vi "Calibrate xtal.vi"(5 "External Attenuation, dB":T8 format="%.2f", 7 "CART TCP Connection In":refnum<k5>, 8 "Error In":errorcluster, 9 "Max Input Power, dBm":T7 format="%.1f", 11 "RFSA Device":T16="RFSA") -> (0 "error out":errorcluster)   [LabVIEW 2012]
doc: "(c) Copyright 2006, National Instruments, Inc. This VI may not be duplicated, sold, or distributed without written consent from National Instruments."
uses:
  <userlib>/niRF/niSystem/SA/Includes/niSYS - RFSA - INC - STYP - Handle.ctl
  <userlib>/niRF/niSystem/SA/Includes/niSYS - SA - INC - STYP - Trigger.ctl
  <userlib>/niRF/niSystem/SA/Includes/niSYS - SA - INC - STYP - Trigger Delay.ctl
  <userlib>/niRF/niSystem/SA/Includes/niSYS - SA - INC - STYP - Timeout.ctl
  <userlib>/niRF/niBasic/SA/Spectrum/Includes/niBASIC - SA - Spectrum - INC - STYP - Averaging.ctl
  <userlib>/niRF/niBasic/SA/Spectrum/Includes/niBASIC - SA - Spectrum - INC - STYP - Measurement.ctl
  <userlib>/niRF/niSystem/SA/Includes/niSYS - SA - INC - STYP - Frequency Reference.ctl
  <userlib>/niRF/niSystem/SA/Includes/niSYS - SA - INC - STYP - External Attenuation.ctl
  <userlib>/niRF/niSystem/SA/Includes/niSYS - SA - INC - STYP - Max Input Power.ctl
  <userlib>/niRF/niSystem/SA/Includes/niSYS - SA - INC - STYP - Center Frequency.ctl
  <userlib>/niRF/niBasic/SA/Spectrum/Includes/niBASIC - SA - Spectrum - INC - STYP - FFT Window.ctl
  <userlib>/niRF/niBasic/SA/Spectrum/Includes/niBASIC - SA - Spectrum - INC - STYP - Measurement RBW.ctl
  <userlib>/niRF/niSystem/SA/Includes/niSYS - SA - INC - STYP - Span.ctl
  <userlib>/niRF/niBasic/SA/Spectrum/Includes/niBASIC - SA - Spectrum - INC - STYP - FFT Size.ctl
  <userlib>/niRF/niBasic/SA/Spectrum/Includes/niBASIC - SA - Spectrum - INC - STYP - Filter Type.ctl
  <userlib>/niRF/niSystem/SA/Includes/niSYS - SA - INC - STYP - Measurement Request.ctl
  <userlib>/niRF/niBasic/SA/Spectrum/Includes/niBASIC - SA - Spectrum - INC - STYP - Measurement Trace Type.ctl
panel:
  out "Array":string[](array[string])
  in  "Filter Type":T1
  in  "FFT Size":T2={"Auto"=enum."On", "Min Pnts/RBW"=3.1, "Window Length"=706, "FFT Length"=1024} {"Min Pnts/RBW" format="%.1f"}
  in  "Span, Hz":T3=1000000.0 format="%^.3e"
  in  "Measurement RBW, Hz":T4={"Auto"=enum."On", "RBW, Hz"=1000000.0} {"RBW, Hz" format="%^.3e"}
  in  "FFT Window":T5
  in  "RFSA Center Frequency, Hz":T6=5500000000.0 format="%^.6e"
  out "Spectrum Graph":T9(graph)={999501953.125, "Time Domain Interval, sec"=4882.8125, "Waveform Measurement Trace"=[-94.58885960127041, -96.86839023376476, -99.44994709212702, -95.73980201325817, -94.85468685558206, -93.89939819937095, -92.96907780368053, -94.62427677362473, -96.00114334271848, -95.0773520951145, -94.62079733063136, -95.66039665905808, -97.26831199401815, -94.4245843897965, -94.11636842862069, -93.58322383773326, -96.15404542236388, -96.24945397470107, -95.50507217914763, -96.54108841377801, -96.20009898290628, -94.5853296471187, -92.45746866418841, -91.28538347271048, -91.87185526400654, -94.56638317616594, -96.80701098668649, -98.3947929158942, -98.51183674015738, -97.19248581591714, -96.81596744977271, -95.42900485531823, -95.06526491233971, -94.58696887517611, -95.97070348701587, -96.12508871585825, -96.44070407370447, -95.79000716907146, -97.40271981045801, -96.56026806674593, -96.63105214105727, -95.37951512730523, -95.0709837906345, -97.57170348129546, -98.65428166191879, -92.85960027957853, -90.69744081914348, -91.78092902523147, -93.01528314210488, -94.00436029202501, -93.35100459361215, -93.65439480062977, -94.03853395069989, -94.46526514886557, -94.89042305851434, -94.67424970039717, -93.63794705250254, -92.45925730447641, -92.65908155014344, -93.60044471338867, -94.45278046002886, -94.14161306416081, -95.1968357622903, -94.78018101642988, -94.3521734655379, -93.66111421566106, -94.84863517357037, -94.5954023919716, -96.31573035476218, -96.10673186698642, -95.71535800929679, -94.23828099215436, -93.52563000159624, -95.57033866863337, -95.53015116793134, -93.56809331780974, -92.7606452725199, -93.57072573308072, -95.32780281550693, -92.86665354898099, -93.1370950166728, -94.12900193004297, -94.87833817452723, -94.72912032302605, -94.17479444496155, -94.72686892886344, -93.6596877329905, -92.66964149507194, -93.08938347771124, -94.20661112927449, -97.92818192608922, -94.73725815144995, -93.72795972831032, -95.83148845299667, -93.96304770180853, -93.50544784378508, -92.44166060977277, -93.27927003206689, -87.23502888503836, -72.11564523212036, -65.2815070033974, -63.751961771120435, -63.76202638288482, -64.94683436227825, -71.0137879230945, -85.10120059441533, -91.83446895184292, -90.61921828145796, -90.72235231920887, -91.03886336724534, -91.42747554368565, -91.50468859500515, -90.91036635524621, -91.23961076459484, -93.16256151029376, -95.66587614800164, -96.70895620214242, -94.44704301225457, -93.34996435212136, -92.18571998503167, -92.8876926563818, -93.5060742547249, -94.69941271506612, -97.92708620913864, -95.25428896670476, -92.62306680566677, -91.3874988202419, -91.85885903026352, -93.43215873965788, -94.90985702146794, -94.99607107512729, -94.53014477422813, -94.84999122998677, -95.93647533060847, -95.05672593509198, -97.64855424631322, -95.46215659926096, -94.67802340702697, -94.36305677166051, -95.093191185747, -95.15591730271399, -94.6393427453004, -95.01042716486224, -93.48932052409448, -93.1088259750116, -95.79379158863588, -94.27401403528606, -94.39185567902642, -95.78566610842289, -96.2278510846579, -97.35096719200405, -94.09028417116734, -93.67455962770373, -92.52661334344788, -92.28656403084389, -93.48717465263262, -95.87262940934153, -96.55075020577934, -96.23995801594376, -95.62432812173306, -95.53325913753295, -95.37316281463609, -96.84726282341614, -96.18759453809396, -92.65258606681302, -91.1549944641086, -91.18877556936353, -91.65922730189286, -92.7088197008887, -93.55252845804509, -93.23891521766758, -93.50579589024103, -93.22879114454076, -93.62878875149401, -94.89920966153908, -94.49841305989179, -94.31891446472981, -93.3315995436115, -92.9576487551588, -94.98762611566268, -97.76488288036198, -96.68686917193047, -95.69013350308543, -95.23811265655995, -95.43343805014592, -96.1176286234256, -98.40428345012647, -97.1939542411557, -93.8709557440311, -92.5732899687502, -93.19402090455232, -93.4806645014271, -92.62376136260087, -93.4169081651324, -95.1135305356191, -95.44327303741449, -95.97664612099189, -95.20918978347628, -93.30477056749844, -92.75514488033883, -92.92596032798458, -94.3147334729053, -95.75765916034278, -97.49920812243585, -93.12822887068018]}
  in  "Frequency Reference":T10={" Reference Source"=enum."On Board Clock", "Frequency, Hz"=10000000.0, "Backplane Source"=enum."None"} {"Frequency, Hz" format="%^.6e"}
  out "Spectrum Measurement":T11={"Peak Amplitude, dBm"=-63.751961771120435, "Peak Frequency, Hz"=999995117.1875, "Number of Points"=256, "Start Frequency, Hz"=999501953.125, "Space Frequency, Hz"=4882.8125} {"Space Frequency, Hz" format="%^.6e"; "Start Frequency, Hz" format="%^.6e"; "Peak Frequency, Hz" format="%^.6e"; "Peak Amplitude, dBm" format="%.2f"}
  in  "Spectrum Averaging":T12={"Averages"=10, "Average State"=enum."On", "Average Mode"=enum."Repeat", "Average Type"=enum."Log"}
  in  "Timeout, sec":T13=10.0 format="%.3f"
  in  "Trigger":T14={"Source"=enum."Immediate", "Edge"=enum."Rising", "Delay, sec"=0.0, "Level, dBm"=-20.0, "Min Quiet Time, sec"=0.0} {"Min Quiet Time, sec" format="%^.2e"; "Level, dBm" format="%.1f"; "Delay, sec" format="%^.2e"}
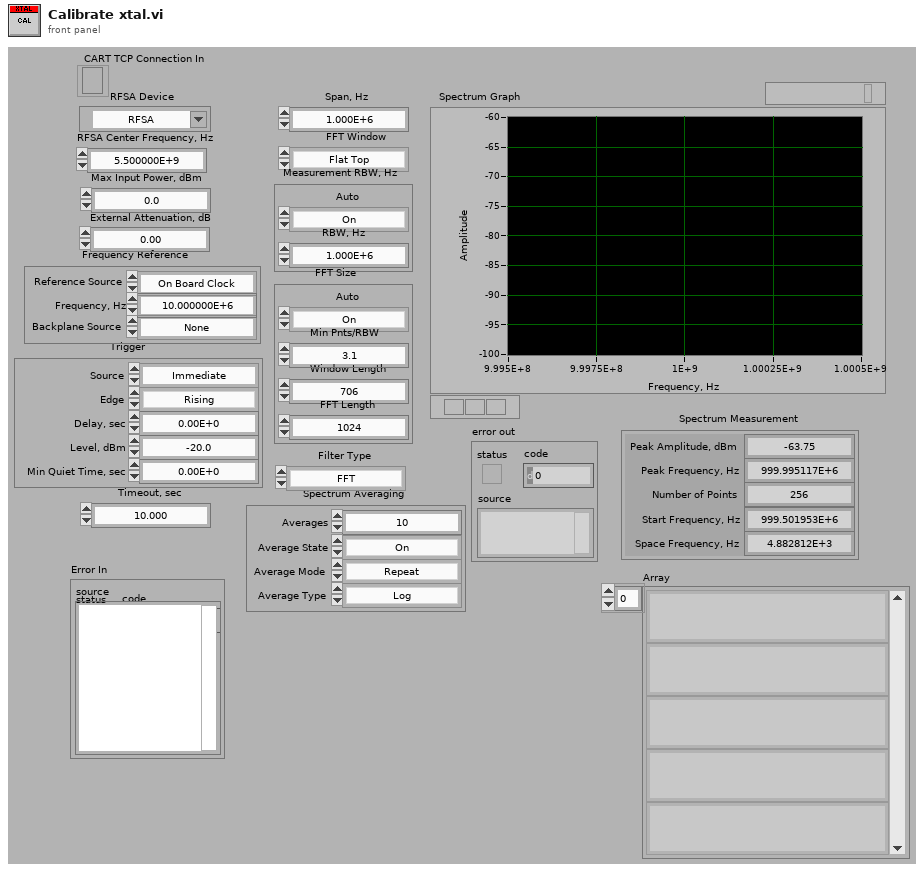
[diagram p1: front panel]
types:
  T1 = typedef "niBASIC - SA - Spectrum - INC - STYP - Filter Type.ctl" = enum16{"FFT", "5-Pole", "Gaussian"}
  T2 = typedef "niBASIC - SA - Spectrum - INC - STYP - FFT Size.ctl" = cluster{"Auto":enum16{"Off", "On"}, "Min Pnts/RBW":dbl, "Window Length":i32, "FFT Length":i32}
  T3 = typedef "niSYS - SA - INC - STYP - Span.ctl" = dbl
  T4 = typedef "niBASIC - SA - Spectrum - INC - STYP - Measurement RBW.ctl" = cluster{"Auto":enum16{"Off", "On"}, "RBW, Hz":dbl}
  T5 = typedef "niBASIC - SA - Spectrum - INC - STYP - FFT Window.ctl" = enum16{"Flat Top", "Uniform", "Hanning", "Hamming", "Gaussian", "Blackman", "Blackman-Harris", "Kaiser-Bessel 70 dB", "Kaiser-Bessel 90 dB", "Kaiser-Bessel 110 dB"}
  T6 = typedef "niSYS - SA - INC - STYP - Center Frequency.ctl" = dbl
  T7 = typedef "niSYS - SA - INC - STYP - Max Input Power.ctl" = dbl
  T8 = typedef "niSYS - SA - INC - STYP - External Attenuation.ctl" = dbl
  T9 = cluster{dbl, "Time Domain Interval, sec":dbl, "Waveform Measurement Trace":dbl[]}
  T10 = typedef "niSYS - SA - INC - STYP - Frequency Reference.ctl" = cluster{" Reference Source":enum16{"On Board Clock", "Ref In", "PXI Clock 10"}, "Frequency, Hz":dbl, "Backplane Source":enum16{"None", "Ref In", "On Board Clock"}}
  T11 = typedef "niBASIC - SA - Spectrum - INC - STYP - Measurement.ctl" = cluster{"Peak Amplitude, dBm":dbl, "Peak Frequency, Hz":dbl, "Number of Points":i32, "Start Frequency, Hz":dbl, "Space Frequency, Hz":dbl}
  T12 = typedef "niBASIC - SA - Spectrum - INC - STYP - Averaging.ctl" = cluster{"Averages":i32, "Average State":enum16{"Off", "On"}, "Average Mode":enum16{"Exponential", "Repeat"}, "Average Type":enum16{"RMS", "Log", "Scalar", "Max", "Min"}}
  T13 = typedef "niSYS - SA - INC - STYP - Timeout.ctl" = dbl
  T14 = typedef "niSYS - SA - INC - STYP - Trigger.ctl" = cluster{"Source":enum16{"Immediate", "External", "Software", "RTSI 0", "RTSI 1", "RTSI 2", "RTSI 3", "RTSI 4", "RTSI 5", "RTSI 6", "RTSI 7", "PFI 0", "PFI 1", "PFI 2", "PXI Star", "Power"}, "Edge":enum16{"Rising", "Falling"}, "Delay, sec":T15, "Level, dBm":dbl, "Min Quiet Time, sec":dbl}
  T15 = typedef "niSYS - SA - INC - STYP - Trigger Delay.ctl" = dbl
  T16 = typedef "niSYS - RFSA - INC - STYP - Handle.ctl" = refnum<k15>
  T17 = typedef "niBASIC - SA - Spectrum - INC - STYP - Measurement Handle.ctl" = refnum<notifier>
  T18 = typedef "niBASIC - SA - Spectrum - INC - STYP - Measurement Trace Type.ctl" = enum16{"Unprocessed I/Q", "Measurements", "Average Spectrum"}
  T19 = typedef "niSYS - SA - INC - STYP - Measurement Request.ctl" = enum16{"Measure", "Fetch", "Initiate"}
  T20 = typedef "niSYS - SA - INC - STYP - Measurement Trace.ctl" = dbl[]
  T21 = typedef "niSYS - SA - INC - STYP - Real Waveform.ctl" = cluster{"x0":dbl, "dx":dbl, "y":dbl[]}
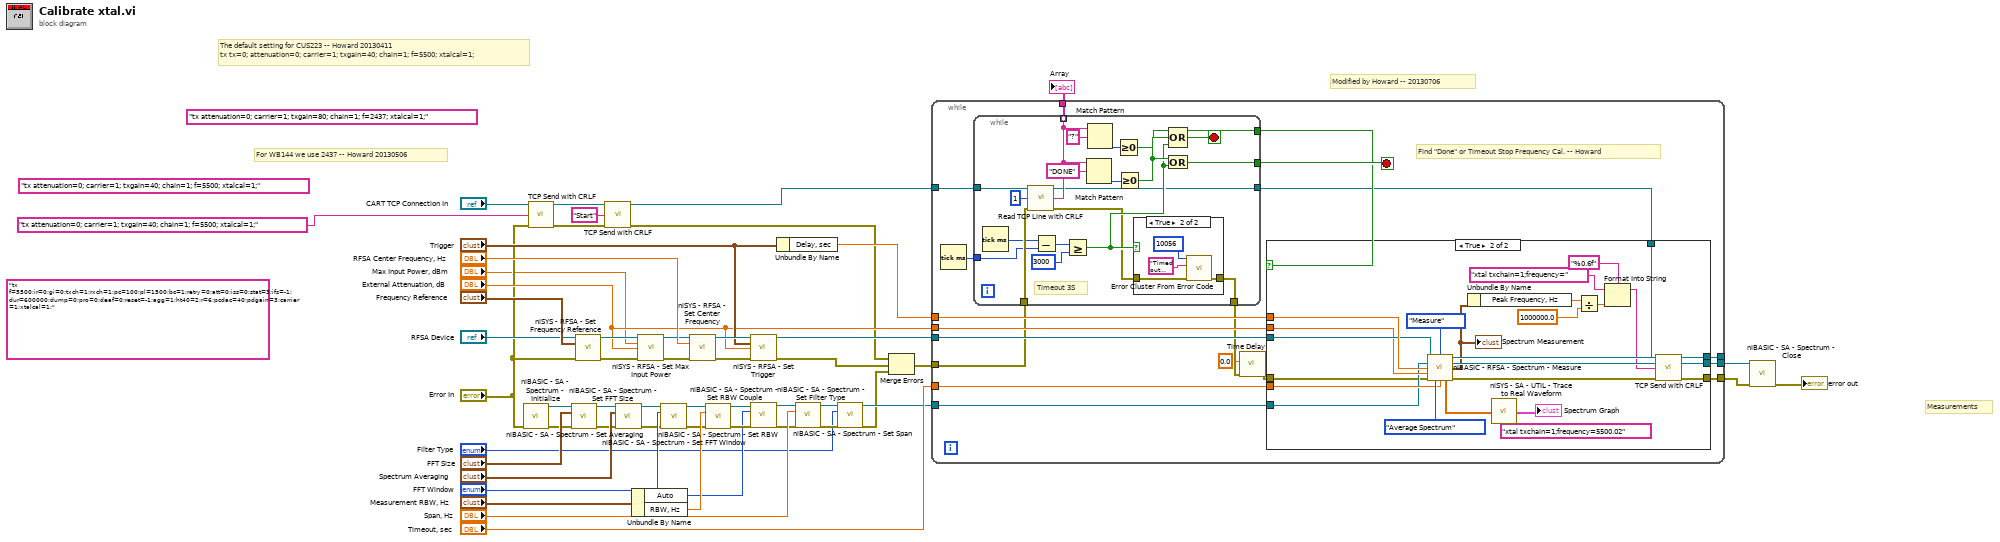
[diagram p0: block diagram]
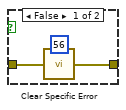
[diagram p2: hidden frame]
diagram:
  (unwired) "tx f=5500;ir=0;gi=0;txch=1;rxch=1;pc=100;pl=1500;bc=1;retry=0;att=0;iss=0;stat=3;ifs=-1;dur=600000;dump=0;pro=0;deaf=0;reset=-1;agg=1;ht40=2;r=6;pcdac=40;pdgain=3;carrier=1;xtalcal=1;"
  (unwired) "tx attenuation=0; carrier=1; txgain=40; chain=1; f=5500; xtalcal=1;" ("data in")
  (unwired) "tx attenuation=0; carrier=1; txgain=80; chain=1; f=2437; xtalcal=1;" ("data in")
  # "Modified by Howard -- 20130706"
  # "For WB144 we use 2437 -- Howard 20130506"
  # "The default setting for CUS223 -- Howard 20130411\ntx tx=0; attenuation=0; carrier=1; txgain=40; chain=1; f=5500; xtalcal=1;"
  # "Measurements"
  n1 = call <userlib>:"niBASIC - SA - Spectrum - Initialize.vi"("error in (no error)"="Error In") -> ("Measurement Handle Out"=w29:T17, "error out"=w30:errorcluster)  [unwired: 1 in, 12 out]
  n2 = call "TCP Send with CRLF.vi"("CART TCP Connection"="CART TCP Connection In", "data in"="tx attenuation=0; carrier=1; txgain=40; chain=1; f=5500; xtalcal=1;", "error IO"="Error In") -> ("CART TCP Connection Out"=w11:refnum<k5>, "error out"=w12:errorcluster)  [unwired: 11 in]
  n3 = call <userlib>:"niBASIC - SA - Spectrum - Set FFT Size.vi"("Measurement Handle In"=w29, "FFT Size"="FFT Size", "error in (no error)"=w30) -> ("Measurement Handle Out"=w43:T17, "error out"=w44:errorcluster)  [unwired: 11 out]
  n4 = call <userlib>:"niSYS - RFSA - Set Frequency Reference.vi"("RFSA Handle In"="RFSA Device", "Frequency Reference"="Frequency Reference", "error in (no error)"="Error In") -> ("RFSA Handle Out"=w32:T16, "error out"=w31:errorcluster)  [unwired: 1 in, 10 out]
  n5 = call "TCP Send with CRLF.vi"("CART TCP Connection"=w11, "data in"="Start", "error IO"=w12) -> ("CART TCP Connection Out"=w9:refnum<k5>, "error out"=w8:errorcluster)  [unwired: 11 in]
  n6 = call <userlib>:"niBASIC - SA - Spectrum - Set Averaging.vi"("Measurement Handle In"=w43, "Averaging"="Spectrum Averaging", "error in (no error)"=w44) -> ("Measurement Handle Out"=w41:T17, "error out"=w42:errorcluster)  [unwired: 11 out]
  n7 = Unbundle By Name("Measurement RBW, Hz") -> ("Auto"=w33:enum16{"Off", "On"}, "RBW, Hz"=w40:dbl)
  n8 = call <userlib>:"niSYS - RFSA - Set Max Input Power.vi"("RFSA Handle In"=w32, "Max Input Power, dBm"="Max Input Power, dBm", "External Attenuation, dB"="External Attenuation, dB", "error in (no error)"=w31) -> ("RFSA Handle Out"=w45:T16, "error out"=w46:errorcluster)  [unwired: 10 out]
  n9 = call <userlib>:"niBASIC - SA - Spectrum - Set FFT Window.vi"("Measurement Handle In"=w41, "FFT Window"="FFT Window", "error in (no error)"=w42) -> ("Measurement Handle Out"=w38:T17, "error out"=w39:errorcluster)  [unwired: 11 out]
  n10 = call <userlib>:"niSYS - RFSA - Set Center Frequency.vi"("RFSA Handle In"=w45, "RFSA Center Frequency, Hz"="RFSA Center Frequency, Hz", "error in (no error)"=w46) -> ("RFSA Handle Out"=w27:T16, "error out"=w28:errorcluster)  [unwired: 11 out]
  n11 = call <userlib>:"niBASIC - SA - Spectrum - Set RBW.vi"("Measurement Handle In"=w38, "RBW, Hz"=w40, "error in (no error)"=w39) -> ("Measurement Handle Out"=w35:T17, "error out"=w37:errorcluster)  [unwired: 11 out]
  n12 = call <userlib>:"niSYS - RFSA - Set Trigger.vi"("RFSA Handle In"=w27, "Trigger"="Trigger", "External Attenuation, dB"="External Attenuation, dB", "error in (no error)"=w28) -> ("RFSA Handle Out"=w24:T16, "error out"=w19:errorcluster)  [unwired: 10 out]
  n13 = call <userlib>:"niBASIC - SA - Spectrum - Set RBW Couple.vi"("Measurement Handle In"=w35, "Auto"=w33, "error in (no error)"=w37) -> ("Measurement Handle Out"=w34:T17, "error out"=w36:errorcluster)  [unwired: 11 out]
  n14 = Unbundle By Name("Trigger") -> ("Delay, sec"=w25:T15)
  n15 = call <userlib>:"niBASIC - SA - Spectrum - Set Span.vi"("Measurement Handle In"=w34, "Span, Hz"="Span, Hz", "error in (no error)"=w36) -> ("Measurement Handle Out"=w18:T17, "error out"=w16:errorcluster)  [unwired: 11 out]
  n16 = call <userlib>:"niBASIC - SA - Spectrum - Set Filter Type.vi"("Measurement Handle In"=w18, "Filter Type"="Filter Type", "error in (no error)"=w16) -> ("Measurement Handle Out"=w17:T17, "error out"=w15:errorcluster)  [unwired: 10 in, 1 out]
  n17 = Merge Errors(w8, w19, w15) -> (w7:errorcluster)
  n18 = while {
    tunnel: w25 -> [w71]
    tunnel: w24 -> [w70]
    tunnel: "External Attenuation, dB" -> [w69]
    tunnel: "Timeout, sec" -> [w68]
    tunnel: [w67] -> _
    tunnel: [w64] -> w4
    tunnel: [w66] -> w21
    tunnel: w17 -> [w65]
    tunnel: w9 -> [w63]
    tunnel: w7 -> [w62]
    tunnel: [w57] -> w3
    stop <- w61 stop-if-true
    # "Find \"Done\" or Timeout Stop Frequency Cal. -- Howard"
    n19 = Tick Count (ms)() -> (millisecond timer value=w58:u32)
    n20 = while {
      tunnel: w63 -> [w86]
      tunnel: w62 -> [w85]
      tunnel: [w79] -> w61
      tunnel: [w76] -> w60
      tunnel: [w75] -> w59
      tunnel: w58 -> [w74]
      tunnel: [w73] -> w57 mode=indexing
      tunnel: [w72] -> w56
      stop <- w81 stop-if-true
      # "Timeout 3S"
      n21 = Tick Count (ms)() -> (millisecond timer value=w84:u32)
      n22 = call "Read TCP Line with CRLF.vi"("TCP Connection In"=w86, "timeout ms (100)"=1, "error in"=w85) -> ("TCP Connection Out"=w72:refnum<k5>, "TCP Line"=w73:string, "error out"=w77:errorcluster)  [unwired: 10 in]
      n23 = Subtract(x=w84, y=w74) -> (x-y=w83:u32)
      n24 = Greater Or Equal?(x=w83, y=u32 3000) -> (x >= y?=w78:bool)
      n25 = Match Pattern(string=w73, regular expression="DONE") -> (offset past match=w91:i32)  [unwired: 1 in, 3 out]
      n26 = Match Pattern(string=w73, regular expression="?") -> (offset past match=w90:i32)  [unwired: 1 in, 3 out]
      n27 = Greater Or Equal To 0?(x=w90) -> (x >= 0?=w75:bool)
      n28 = Greater Or Equal To 0?(x=w91) -> (x >= 0?=w80:bool)
      n29 = case shown="True" w78 {
        tunnel: w77 -> [w93 w98]
        tunnel: [w92 w96] -> w76
        frame False {
          n30 = call "Clear Specific Error.vi"("Specific Error Number (0: none)"=56 ("Specific Error Number"), "error in"=w93) -> ("error out"=w92:errorcluster)  [unwired: 12 in, 1 out]
        }
        frame True {
          n31 = call <vilib>:"Error Cluster From Error Code.vi"("error in (no error)"=w98, "error message (\"\")"="Timed out waiting for desired response." ("format string"), "error code (0)"=10056) -> ("error out"=w96:errorcluster)  [unwired: 6 in]
        }
      }
      n32 = Compound Arithmetic op=OR(w75, w80, w78) -> (w81:bool)
      n33 = Compound Arithmetic op=OR(w80, w78) -> (w79:bool)
    }
    n34 = call "Time Delay"("error in (no error)"=w60, "Delay Time (s)"=0.0) -> ("error out"=w55:errorcluster)  [unwired: 9 in]
    n35 = case shown="True" w59 {
      tunnel: w71 -> [_ w123]
      tunnel: w70 -> [w100 w122]
      tunnel: w69 -> [_ w121]
      tunnel: w68 -> [_ w118]
      tunnel: [w100 w117] -> w67
      tunnel: [w101 w116] -> w66
      tunnel: w65 -> [w101 w115]
      tunnel: [w99 w109] -> w64
      tunnel: w55 -> [w99 w106]
      tunnel: w56 -> [_ w105]
      frame False {
      }
      frame True {
        (unwired) "xtal txchain=1;frequency=5500.02" ("format string")
        n36 = call <userlib>:"niBASIC - RFSA - Spectrum - Measure.vi"("RFSA Handle In"=w122, "Measurement Request"=niSYS_-_SA_-_INC_-_STYP_-_Measurement_Request."Measure", "Measurement Handle In"=w115, "Trigger Delay, sec"=w123, "External Attenuation, dB"=w121, "error in (no error)"=w106, "Measurement Trace Type"=niBASIC_-_SA_-_Spectrum_-_INC_-_STYP_-_Measurement_Trace_Type."Average Spectrum", "Timeout, sec"=w118) -> ("RFSA Handle Out"=w117:T16, "Measurement Handle Out"=w116:T17, "Measurement"=w114:T11, "Measurement Trace"=w107:T20, "error out"=w110:errorcluster)  [unwired: 3 out]
        "Spectrum Measurement" <- w114
        n37 = Unbundle By Name(w114) -> ("Peak Frequency, Hz"=w113:dbl)
        n38 = call <userlib>:"niSYS - SA - UTIL - Trace to Real Waveform.vi"("Measurement Trace"=w107) -> ("Signal"=→"Spectrum Graph":T21)
        n39 = Divide(x=w113, y=1000000.0) -> (x/y=w112:dbl)
        n40 = Format Into String(format string="%0.6f", initial string="xtal txchain=1;frequency=" ("format string"), w112) -> (resulting string=w102:string)  [unwired: 1 in, 1 out]
        n41 = call "TCP Send with CRLF.vi"("CART TCP Connection"=w105, "data in"=w102, "error IO"=w110) -> ("error out"=w109:errorcluster)  [unwired: 11 in, 1 out]
      }
    }
  }
  "Array" <- w3
  n42 = call <userlib>:"niBASIC - SA - Spectrum - Close.vi"("Measurement Handle In"=w21, "error in (no error)"=w4) -> ("error out"=→"error out":errorcluster)  [unwired: 13 out]
